vi "fgt get pressure Channel Count.vi"(8 "error in (no error)":errorcluster) -> (0 "error out":errorcluster, 3 "nbPChan out":u32)   [LabVIEW 2016, in "fgt_SDK.lvlib"]
doc: "Get total number of initialized pressure channels. It is the sum of all MFCS, MFCS-EZ and FlowEZ pressure controllers"
uses:
  fgt_SDK.lvlib
  dlls/fgt_SDK_32.dll
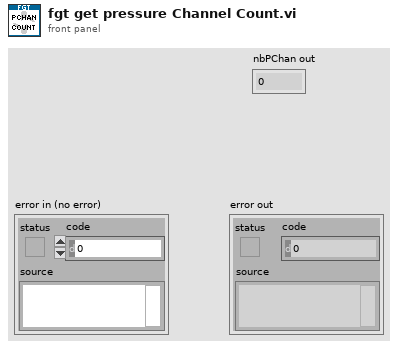
[diagram p1: front panel]
types:
  T1 = typedef "fgt_SDK.lvlib/fgt_STATUS_INFO.ctl" = cluster{"InstrType":T2, "instrSN":u16, "errorCode":u8, "infoCode":u8, "detail":string}
  T2 = typedef "fgt_SDK.lvlib/fgt_INSTRUMENT_TYPE.ctl" = enum32{"None", "MFCS", "MFCS_EZ", "FRP", "LineUP"}
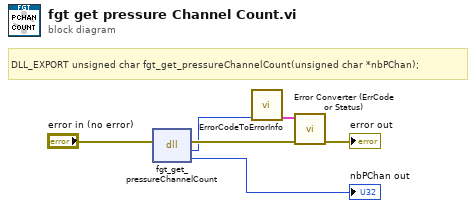
[diagram p0: block diagram]
diagram:
  # "DLL_EXPORT unsigned char fgt_get_pressureChannelCount(unsigned char *nbPChan);"
  n1 = dll-call lib="PTH2Zabs D\nMes DocumentsDéveloppementFluigentSDKsfgt-sdk-labviewdllsfgt_SDK_*.*" fn="fgt_get_pressureChannelCount"(error in="error in (no error)") -> (error out=w5:errorcluster, "return type"=w2:u8, "nbPChan"=→"nbPChan out":u8)  [unwired: 3 in, 1 out]
  n2 = call "ErrorCodeToErrorInfo.vi"("return type"=w2) -> ("StatusInfo"=w3:T1)  [unwired: 10 in]
  n3 = call "Error Converter (ErrCode or Status).vi"("error in (no error)"=w5, "StatusInfo"=w3) -> ("error out"=→"error out":errorcluster)  [unwired: 9 in]
